vi "get_material_name.vi"(8 "error in (no error)":errorcluster, 10 "Material number":u8, 11 "VISA resource name":refnum<visa-resource-name>) -> (0 "error out":errorcluster, 2 "Material name":string, 3 "VISA resource name out":refnum<visa-resource-name>)   [LabVIEW 2018]
doc: "Update the name of an output."
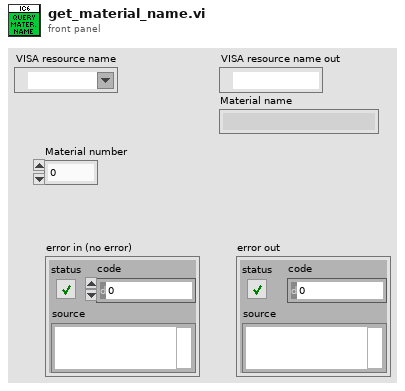
[diagram p1: front panel]
types:
  T1 = enum16{"Source", "General", "Input name", "Process name", "Logic", "Material", "Material name", "Output name", "Process", "Sensor", "Output type", "User message", "Layer", ""}
  T2 = enum16{"Hello", "Query", "Remote action", "Status", "Update"}
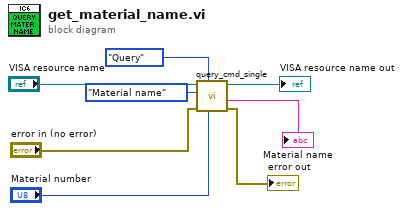
[diagram p0: block diagram]
diagram:
  n1 = call "query_cmd_single.vi"("Parameter"="Material number", "Command group"=T2."Query", "error in (no error)"="error in (no error)", "Command subgroup"=T1."Material name", "VISA resource name"="VISA resource name") -> ("error out"=→"error out":errorcluster, "formatted response"=→"Material name":string, "VISA resource name out"=→"VISA resource name out":refnum<visa-resource-name>)  [unwired: 2 in, 2 out]
